vi "CLSUIP_Write Future Parent ProjectItem.vi"(8 "error in (no error)":errorcluster, 10 "Future Parent ProjectItem":refnum<vi>, 11 "VIRetooler in":refnum<class "VIRetooler.lvclass">) -> (0 "error out":errorcluster, 3 "VIRetooler out":refnum<class "VIRetooler.lvclass">)   [LabVIEW 2021, in "MemberVICreation.lvlib" / "VIRetooler.lvclass"]
uses:
  <resource>/Framework/Providers/LVClassLibrary/NewAccessors/VIRetooler/VIRetooler.lvclass
  <resource>/Framework/Providers/LVClassLibrary/NewAccessors/VIRetooler/VIRetooler.lvclass/VIRetooler.ctl
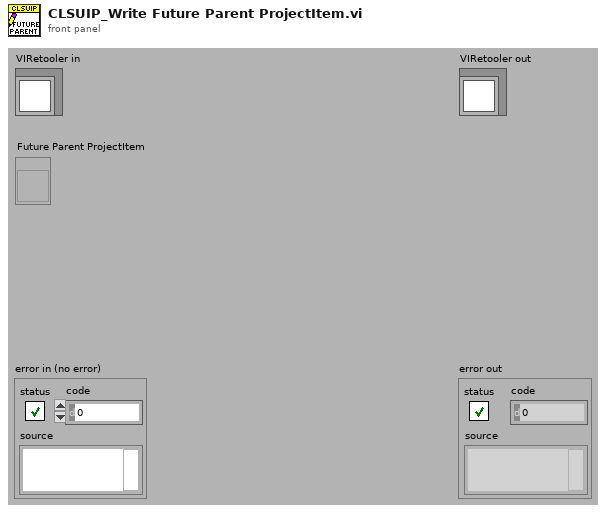
[diagram p1: front panel]
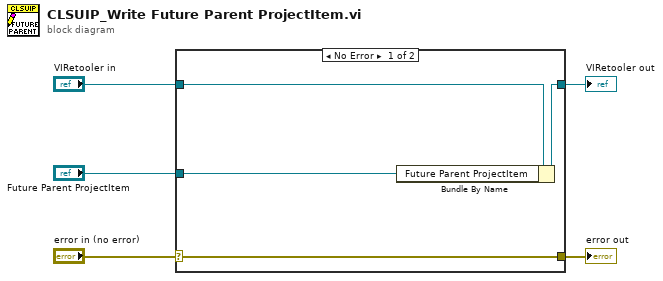
[diagram p0: block diagram]
diagram:
  n1 = case shown="No Error" "error in (no error)" {
    selector: "error in (no error)" -> [w9 w10]
    tunnel: [w9 w10] -> w4
    tunnel: [w7 w11] -> w2
    tunnel: "VIRetooler in" -> [w8 w11]
    tunnel: "Future Parent ProjectItem" -> [w6 _]
    frame No Error {
      n2 = Bundle By Name(cluster=w8, "Future Parent ProjectItem"=w6) -> (w7:refnum<class "VIRetooler.lvclass">)
    }
    frame Error {
    }
  }
  "error out" <- w4
  "VIRetooler out" <- w2
